vi "InsertSingleData.vi"(6 "String In":string, 8 "error in (no error)":errorcluster, 9 "Col":i32, 10 "Row":i32, 11 "Table in":refnum<vi>) -> (0 "error out":errorcluster)   [LabVIEW 2017]
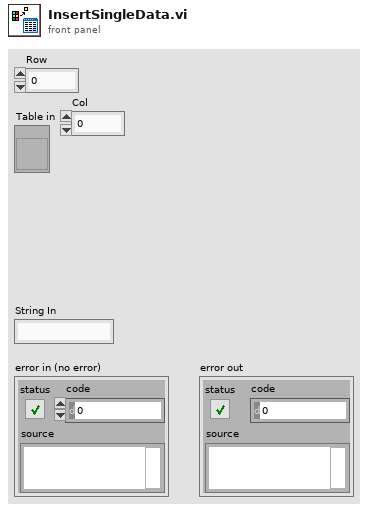
[diagram p1: front panel]
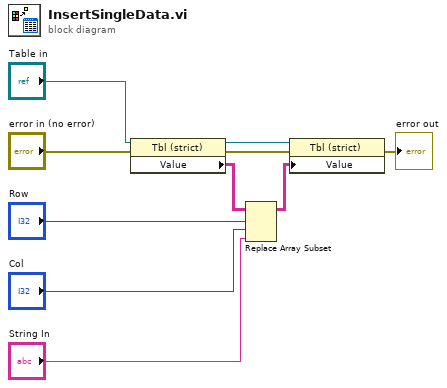
[diagram p0: block diagram]
diagram:
  n1 = property class="Tbl (strict)"(reference="Table in", error in="error in (no error)") -> (reference out=w8:refnum<vi>, error out=w4:errorcluster, "Value"=w5:string[][])
  n2 = Replace Array Subset(array=w5, new element="String In", index (row)="Row", index (col)="Col") -> (w6:string[][])
  n3 = property class="Tbl (strict)"(reference=w8, error in=w4, "Value"=w6) -> (error out=→"error out":errorcluster)  [unwired: 1 out]
